vi "Parity Determiner.vi"(10 "Array":dbl[](array[numeric])) -> (2 "Output Cluster":T1)   [LabVIEW 2017]
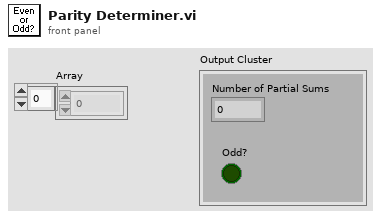
[diagram p1: front panel]
types:
  T1 = cluster{"Number of Partial Sums":i32, "Odd?":bool}
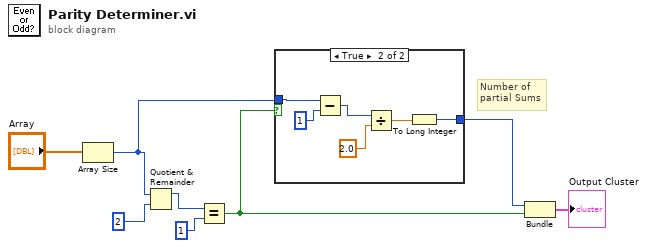
[diagram p0: block diagram]
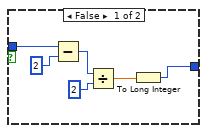
[diagram p2: hidden frame]
diagram:
  # "Number of \npartial Sums"
  n1 = Array Size(array="Array") -> (size(s)=w3:i32)
  n2 = Quotient & Remainder(x=w3, y=2) -> (x-y*floor(x/y)=w5:i32)  [unwired: 1 out]
  n3 = Equal?(x=w5, y=1) -> (x = y?=w4:bool)
  n4 = case shown="True" w4 {
    tunnel: w3 -> [w12 w19]
    tunnel: [w9 w15] -> w2
    frame False {
      n5 = Subtract(x=w12, y=2) -> (x-y=w11:i32)
      n6 = Divide(x=w11, y=2) -> (x/y=w10:dbl)
      n7 = To Long Integer(number=w10) -> (32bit integer=w9:i32)
    }
    frame True {
      n8 = Subtract(x=w19, y=1) -> (x-y=w17:i32)
      n9 = Divide(x=w17, y=2.0) -> (x/y=w16:dbl)
      n10 = To Long Integer(number=w16) -> (32bit integer=w15:i32)
    }
  }
  n11 = Bundle(w2, w4) -> (→"Output Cluster":cluster{i32, bool})  [unwired: 1 in]
